vi "Global Data.vi"() -> ()   [LabVIEW 2015]
panel:
  out "Iterations":ext
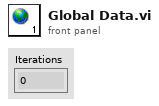
[diagram p1: front panel]
diagram:
